vi "Get norm to um scaling .vi"(8 "error in (no error)":errorcluster, 11 "Current Objective":string) -> (0 "error out":errorcluster, 1 "Objective HW Settings":T1, 2 "X_norm to um_scaling":dbl, 3 "Z_norm to um_scaling":dbl)   [LabVIEW 2020]
uses:
  Typedefs/Objective Config.ctl
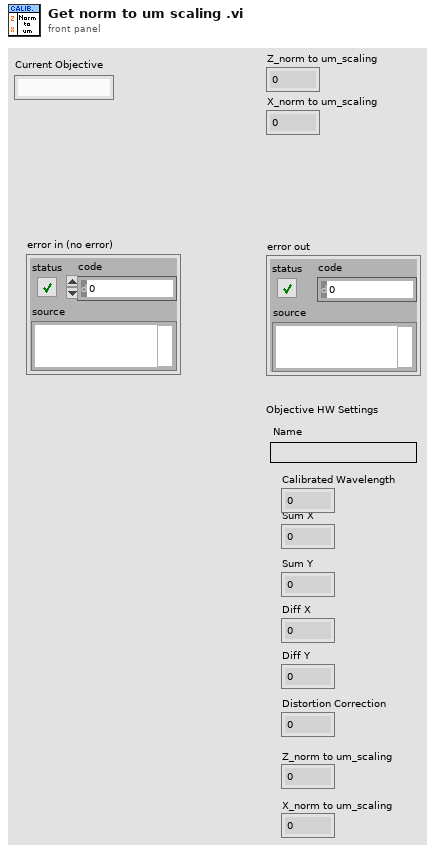
[diagram p1: front panel]
types:
  T1 = typedef "Objective Config.ctl" = cluster{"Name":string, "Sum X":dbl, "Sum Y":dbl, "Diff X":dbl, "Diff Y":dbl, "Distortion Correction":dbl, "Z_norm to um_scaling":dbl, "X_norm to um_scaling":dbl, "Calibrated Wavelength":dbl}
  T2 = enum16{"Initialise", "Load from file", "Save to file", "Read", "Write"}
  T3 = typedef "Calibration config.ctl" = cluster{"Current Objective":string, "Objective Settings":T1[], "PreChirper Values Preset ?":bool, "PreChirper Settings":T4[], "PreChirper Constants":T5}
  T4 = typedef "Prechirper Cal Config.ctl" = cluster{"Wavelength":i32, "Prism 1":i32, "Prism 2":i32}
  T5 = typedef "PreChirper constants.ctl" = cluster{"a 1":i32, "b 1":i32, "c 1":i32, "a 2":i32, "b 2":i32, "c 2":i32, "lmin":i32, "lmax":i32}
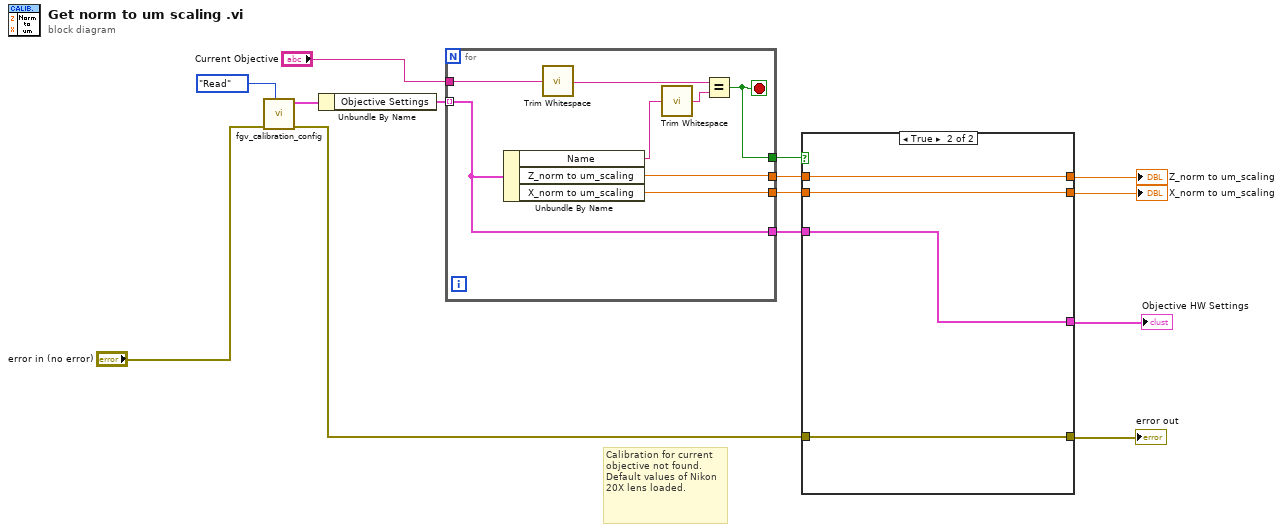
[diagram p0: block diagram]
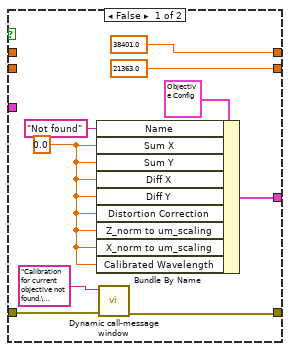
[diagram p2: hidden frame]
diagram:
  # "Calibration for current objective not found.\nDefault values of Nikon 20X lens loaded."
  n1 = call "fgv_calibration_config.vi"("Cal config ops"=T2."Read", "error in (no error)"="error in (no error)") -> ("error out"=w5:errorcluster, "Config cluster OUT"=w13:T3)  [unwired: 7 in, 1 out]
  n2 = Unbundle By Name(w13) -> ("Objective Settings"=w12:T1[])
  n3 = for {
    tunnel: "Current Objective" -> [w22]
    tunnel: w12 -> [w15] mode=indexing
    tunnel: [w18] -> w10
    tunnel: [w17] -> w8
    tunnel: [w16] -> w11
    tunnel: [w15] -> w2
    stop <- w16 stop-if-true
    n4 = Unbundle By Name(w15) -> ("Name"=w21:string, "Z_norm to um_scaling"=w18:dbl, "X_norm to um_scaling"=w17:dbl)
    n5 = call <vilib>:"Trim Whitespace.vi"("string"=w22) -> ("trimmed string"=w19:string)  [unwired: 1 in]
    n6 = call <vilib>:"Trim Whitespace.vi"("string"=w21) -> ("trimmed string"=w20:string)  [unwired: 1 in]
    n7 = Equal?(x=w19, y=w20) -> (x = y?=w16:bool)
  }
  n8 = case shown="True" w11 {
    tunnel: w10 -> [_ w35]
    tunnel: [38401.0 ("Z_norm to um_scaling") w35] -> w9
    tunnel: w8 -> [_ w34]
    tunnel: [21363.0 ("X_norm to um_scaling") w34] -> w7
    tunnel: w5 -> [w29 w33]
    tunnel: [w28 w33] -> w4
    tunnel: w2 -> [_ w32]
    tunnel: [w25 w32] -> w1
    frame False {
      w23 = 0.0 ("Sum X")
      n9 = Bundle By Name(cluster=T1 {"Name"="", "Sum X"=0.0, "Sum Y"=0.0, "Diff X"=0.0, "Diff Y"=0.0, "Distortion Correction"=0.0, "Z_norm to um_scaling"=0.0, "X_norm to um_scaling"=0.0, "Calibrated Wavelength"=0.0} ("Objective HW Settings"), "Name"="Not found", "Sum X"=w23, "Sum Y"=w23, "Diff X"=w23, "Diff Y"=w23, "Distortion Correction"=w23, "Z_norm to um_scaling"=w23, "X_norm to um_scaling"=w23, "Calibrated Wavelength"=w23) -> (w25:T1)
      n10 = call "Dynamic call-message window.vi"("error in (no error)"=w29, "Message"="Calibration for current objective not found.\nDefault values of Nikon 20X lens loaded. ") -> ("error out"=w28:errorcluster)  [unwired: 9 in]
    }
    frame True {
    }
  }
  "Z_norm to um_scaling" <- w9
  "X_norm to um_scaling" <- w7
  "error out" <- w4
  "Objective HW Settings" <- w1
